vi "create black image in first folder.vi"(8 "error in (no error)":errorcluster, 10 "path":path, 11 "TomoConversion in":refnum<class "TomoConversion.lvclass">) -> (0 "error out":errorcluster, 3 "TomoConversion out":refnum<class "TomoConversion.lvclass">)   [LabVIEW 2012, in "TomoConversion.lvclass"]
uses:
  TomoConversion.lvclass
  TomoConversion.lvclass/TomoConversion.ctl
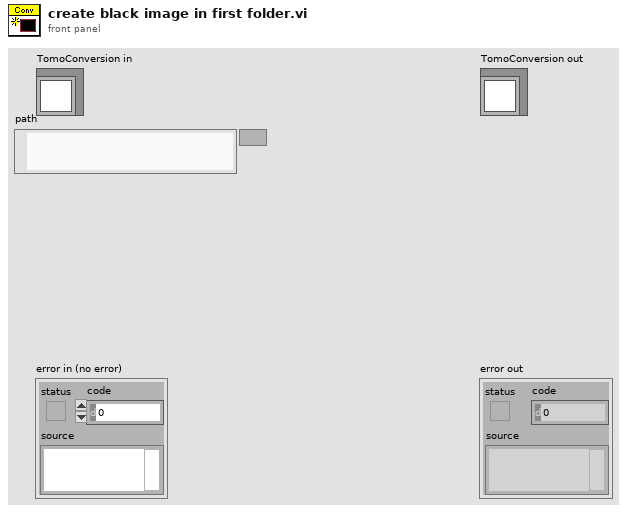
[diagram p1: front panel]
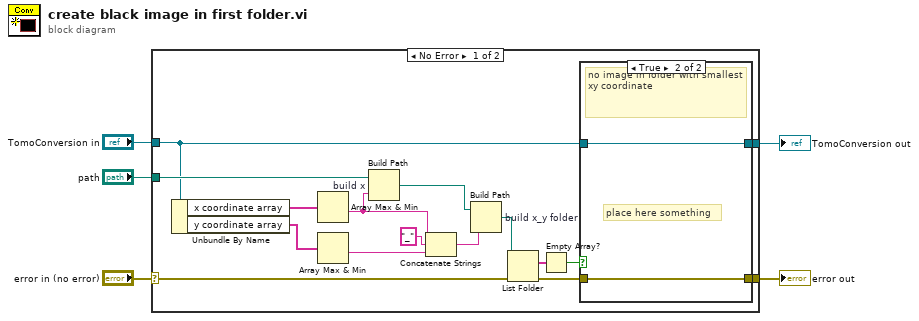
[diagram p0: block diagram]
diagram:
  n1 = case shown="No Error" "error in (no error)" {
    selector: "error in (no error)" -> [w13 w27]
    tunnel: [w6 w27] -> w4
    tunnel: [w7 w26] -> w2
    tunnel: "TomoConversion in" -> [w9 w26]
    tunnel: "path" -> [w16 _]
    frame No Error {
      n2 = Unbundle By Name(w9) -> ("x coordinate array"=w21:string[], "y coordinate array"=w20:string[])
      n3 = Array Max & Min(array=w21) -> (min value=w15:string)  [unwired: 3 out]
      n4 = Array Max & Min(array=w20) -> (min value=w17:string)  [unwired: 3 out]
      n5 = Build Path "build x"(base path=w16, name or relative path=w15) -> (appended path=w14:path)
      n6 = Concatenate Strings(w15, "_" ("string"), w17) -> (w19:string)
      n7 = Build Path "build x_y folder"(base path=w14, name or relative path=w19) -> (appended path=w12:path)
      n8 = List Folder(path=w12, error in=w13) -> (filenames=w11:string[], error out=w10:errorcluster)  [unwired: 2 in, 2 out]
      n9 = Empty Array?(array=w11) -> (empty?=w8:bool)
      n10 = case shown="True" w8 {
        tunnel: w10 -> [w22 w24]
        tunnel: w9 -> [w23 w25]
        tunnel: [w23 w25] -> w7
        tunnel: [w22 w24] -> w6
        frame False {
        }
        frame True {
          # "place here something"
          # "no image in folder with smallest xy coordinate"
        }
      }
    }
    frame Error {
    }
  }
  "error out" <- w4
  "TomoConversion out" <- w2
